vi "Write configuration.vi"(8 "error in (no error)":errorcluster, 11 "DAQMH121119OrcaFlash in":refnum<class "DAQOrcaFlash.lvclass">) -> (0 "error out":errorcluster, 3 "DAQMH121119OrcaFlash out":refnum<class "DAQOrcaFlash.lvclass">)   [LabVIEW 2012, in "DAQOrcaFlash.lvclass"]
doc: "Writes the configuration cluster into the configuration file. Configuration file is XML-based. It's name is <component ID>.xml"
uses:
  DAQOrcaFlash.lvclass
  <vilib>/Distrio/Murmex/Murmex/Murmex.lvclass
  DAQOrcaFlash.lvclass/DAQOrcaFlash.ctl
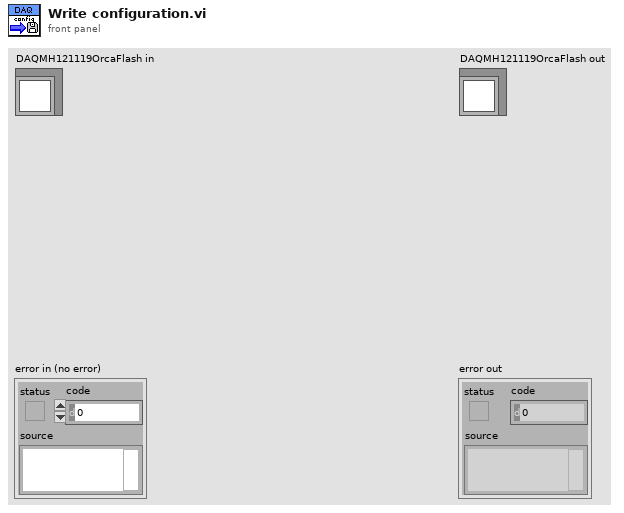
[diagram p1: front panel]
types:
  T1 = typedef "DAQOrcaFlash.lvclass/configuration_cluster.ctl" = cluster{"filepath":path, "Trigger source":T2, "Trigger mode":T3, "Sensor mode":T4, "Read out direction":T5, "Output trigger type":T6, "Output trigger source":T7, "Output trigger period":sgl[unit], "start_stop_targets":string[], "Output trigger connector":T8, "Stack component":string, "Tomo component":string, "auxiliary folders paths":path[], "maximum window size":i32, "final conversion folder":path, "Output trigger polarity":T9, "Input trigger polarity":T9, "Autofocus component":string}
  T2 = typedef "DAQOrcaFlash.lvclass/trigger_source.ctl" = sgl
  T3 = typedef "DAQOrcaFlash.lvclass/trigger_mode.ctl" = sgl
  T4 = typedef "DAQOrcaFlash.lvclass/sensor_mode.ctl" = sgl
  T5 = typedef "DAQOrcaFlash.lvclass/read out direction.ctl" = sgl
  T6 = typedef "DAQOrcaFlash.lvclass/output trigger type.ctl" = sgl
  T7 = typedef "DAQOrcaFlash.lvclass/output trigger source.ctl" = sgl
  T8 = typedef "DAQOrcaFlash.lvclass/connector.ctl" = enum32{"1", "2", "3"}
  T9 = typedef "DAQOrcaFlash.lvclass/trigger_polarity.ctl" = sgl
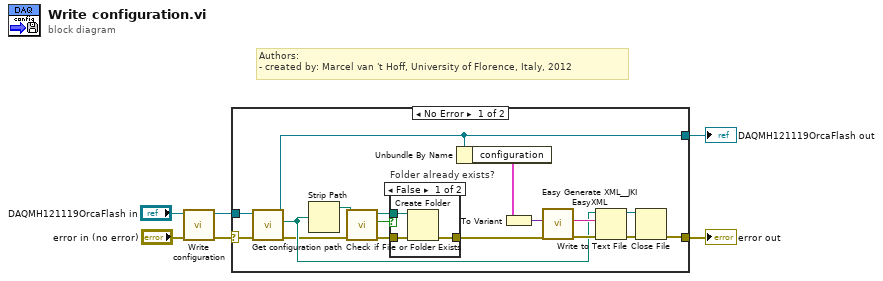
[diagram p0: block diagram]
diagram:
  # "Authors: \n- created by: Marcel van 't Hoff, University of Florence, Italy, 2012"
  n1 = call-parent "Write configuration.vi"("error in (no error)"="error in (no error)", "Murmex in"="DAQMH121119OrcaFlash in") -> ("error out"=w4:errorcluster, "Murmex out"=w2:refnum<class "DAQOrcaFlash.lvclass">)  [unwired: 8 in]
  n2 = case shown="No Error" w4 {
    selector: w4 -> [w9 w29]
    tunnel: [w21 w29] -> w3
    tunnel: [w7 w28] -> w1
    tunnel: w2 -> [w8 w28]
    frame No Error {
      n3 = call <vilib>:"Get configuration path.vi"("error in (no error)"=w9, "Murmex in"=w8) -> ("error out"=w12:errorcluster, "configuration path"=w15:path, "Murmex out"=w7:refnum<class "DAQOrcaFlash.lvclass">)  [unwired: 7 in]
      n4 = Strip Path(path=w15) -> (stripped path=w14:path)  [unwired: 1 out]
      n5 = call <vilib>:"Check if File or Folder Exists.vi"("error in (no error)"=w12, "path"=w14) -> ("error out"=w11:errorcluster, "file or folder exists?"=w10:bool, "dup path"=w13:path)  [unwired: 7 in]
      n6 = case "Folder already exists?" shown="False" w10 {
        tunnel: [w26 w27] -> w16
        tunnel: w13 -> [w25 _]
        tunnel: w11 -> [w24 w27]
        frame False {
          n7 = Create Folder(path (use dialog)=w25, error in=w24) -> (error out=w26:errorcluster)  [unwired: 1 in, 2 out]
        }
        frame True {
        }
      }
      n8 = Unbundle By Name(w7) -> ("configuration"=w19:T1)
      n9 = To Variant(anything=w19) -> (Variant=w20:variant)
      n10 = call <vilib>:"Easy Generate XML__JKI EasyXML.vi"("error in (no error)"=w16, "LabVIEW Data"=w20) -> ("error out"=w18:errorcluster, "XML String"=w17:string)  [unwired: 8 in]
      n11 = Write to Text File(file (use dialog)=w15, text=w17, error in=w18) -> (refnum out=w23:refnum<file>, error out=w22:errorcluster)  [unwired: 1 in, 1 out]
      n12 = Close File(refnum=w23, error in=w22) -> (error out=w21:errorcluster)  [unwired: 1 out]
    }
    frame Error {
    }
  }
  "error out" <- w3
  "DAQMH121119OrcaFlash out" <- w1
